vi "Enclose in Structure - Offset Structure.vi"(10 "Structure Type":T1, 11 "MasterRect in":T2) -> (3 "MasterRect out":T2)   [LabVIEW 2020]
uses:
  <vilib>/Utility/miscctls.llb/LVRectTypeDef.ctl
  Enclose in Structure - Structure Type.ctl
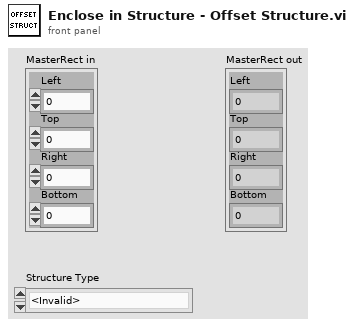
[diagram p1: front panel]
types:
  T1 = typedef "Enclose in Structure - Structure Type.ctl" = enum16{"<Invalid>", "For Loop", "While Loop", "Timed Loop", "Timed Sequence", "Case Structure", "Event Structure", "In Place Element Structure", "Flat Sequence", "Diagram Disable Structure", "Conditional Disable Structure", "Type Specialization Structure"}
  T2 = typedef "LVRectTypeDef.ctl" = cluster{"Left":i16, "Top":i16, "Right":i16, "Bottom":i16}
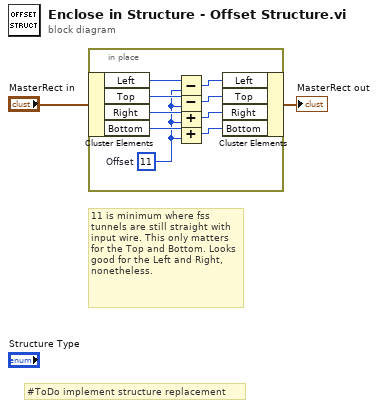
[diagram p0: block diagram]
diagram:
  # "#ToDo implement structure replacement"
  # "11 is minimum where fss tunnels are still straight with input wire. This only matters for the Top and Bottom. Looks good for the Left and Right, nonetheless."
  n1 = in-place {
    w3 = i16 11  # Offset
    n2 = in-place-cluster #1("MasterRect in") -> ("Left"=w11:i16, "Top"=w10:i16, "Right"=w9:i16, "Bottom"=w8:i16)
    n3 = Subtract(x=w11, y=w3) -> (x-y=w7:i16)
    n4 = Subtract(x=w10, y=w3) -> (x-y=w6:i16)
    n5 = Add(x=w9, y=w3) -> (x+y=w5:i16)
    n6 = Add(x=w8, y=w3) -> (x+y=w4:i16)
    n7 = in-place-cluster #1("Left"=w7, "Top"=w6, "Right"=w5, "Bottom"=w4) -> (→"MasterRect out":T2)
  }
